vi "ElephantMultThread.vi"   [LabVIEW 2014]
uses:
  <vilib>/NXT/Block Support/NXT_ButtonSelector.ctl
  <vilib>/NXT/Block Support/NXT_InputPort.ctl
  <vilib>/NXT/Block Support/NXT_OutputPort.ctl
  <vilib>/NXT/Dual Mode Library/Waits/Wait_EV3_Color_Red_Less.vi
  <vilib>/NXT/Dual Mode Library/Waits/Wait_EV3_Color_Red_Greater.vi
  <vilib>/NXT/Dual Mode Library/Sound/PlaySoundFile.vi
  <vilib>/NXT/Dual Mode Library/Waits/Wait_Btn_Release.vi
  <vilib>/NXT/Dual Mode Library/Waits/Wait_Btn_Press.vi
  <vilib>/NXT/NXTIO Xnodes/NXTIONodeSubVIs/NXTStopMotors.vi
  <vilib>/NXT/NXTIO Xnodes/NXTIONodeSubVIs/NXTMoveMotors.vi
  <vilib>/NXT/Dual Mode Library/Waits/Wait_LetGo.vi
  <vilib>/NXT/Dual Mode Library/Waits/Wait_Touch.vi
  <vilib>/NXT/NXTIO Xnodes/NXTIONodeSubVIs/LEGOResetMotors.vi
  <vilib>/NXT/NXTIO Xnodes/AddressXNode/NXTIOAddress.xnode
  <vilib>/NXT/NXTIO Xnodes/NXTIOXNode/NXTIO.xnode
  <vilib>/NXT/Subs/LVHSConnector.ctl
  <vilib>/NXT/LegoClasses/BrickReference/BrickReference.lvclass
types:
  T1 = typedef "NXT_InputPort.ctl" = u32
  T2 = typedef "NXT_ButtonSelector.ctl" = u16
  T3 = typedef "NXT_OutputPort.ctl" = u8
  T4 = typedef "LVHSConnector.ctl" = refnum<class "BrickReference.lvclass">
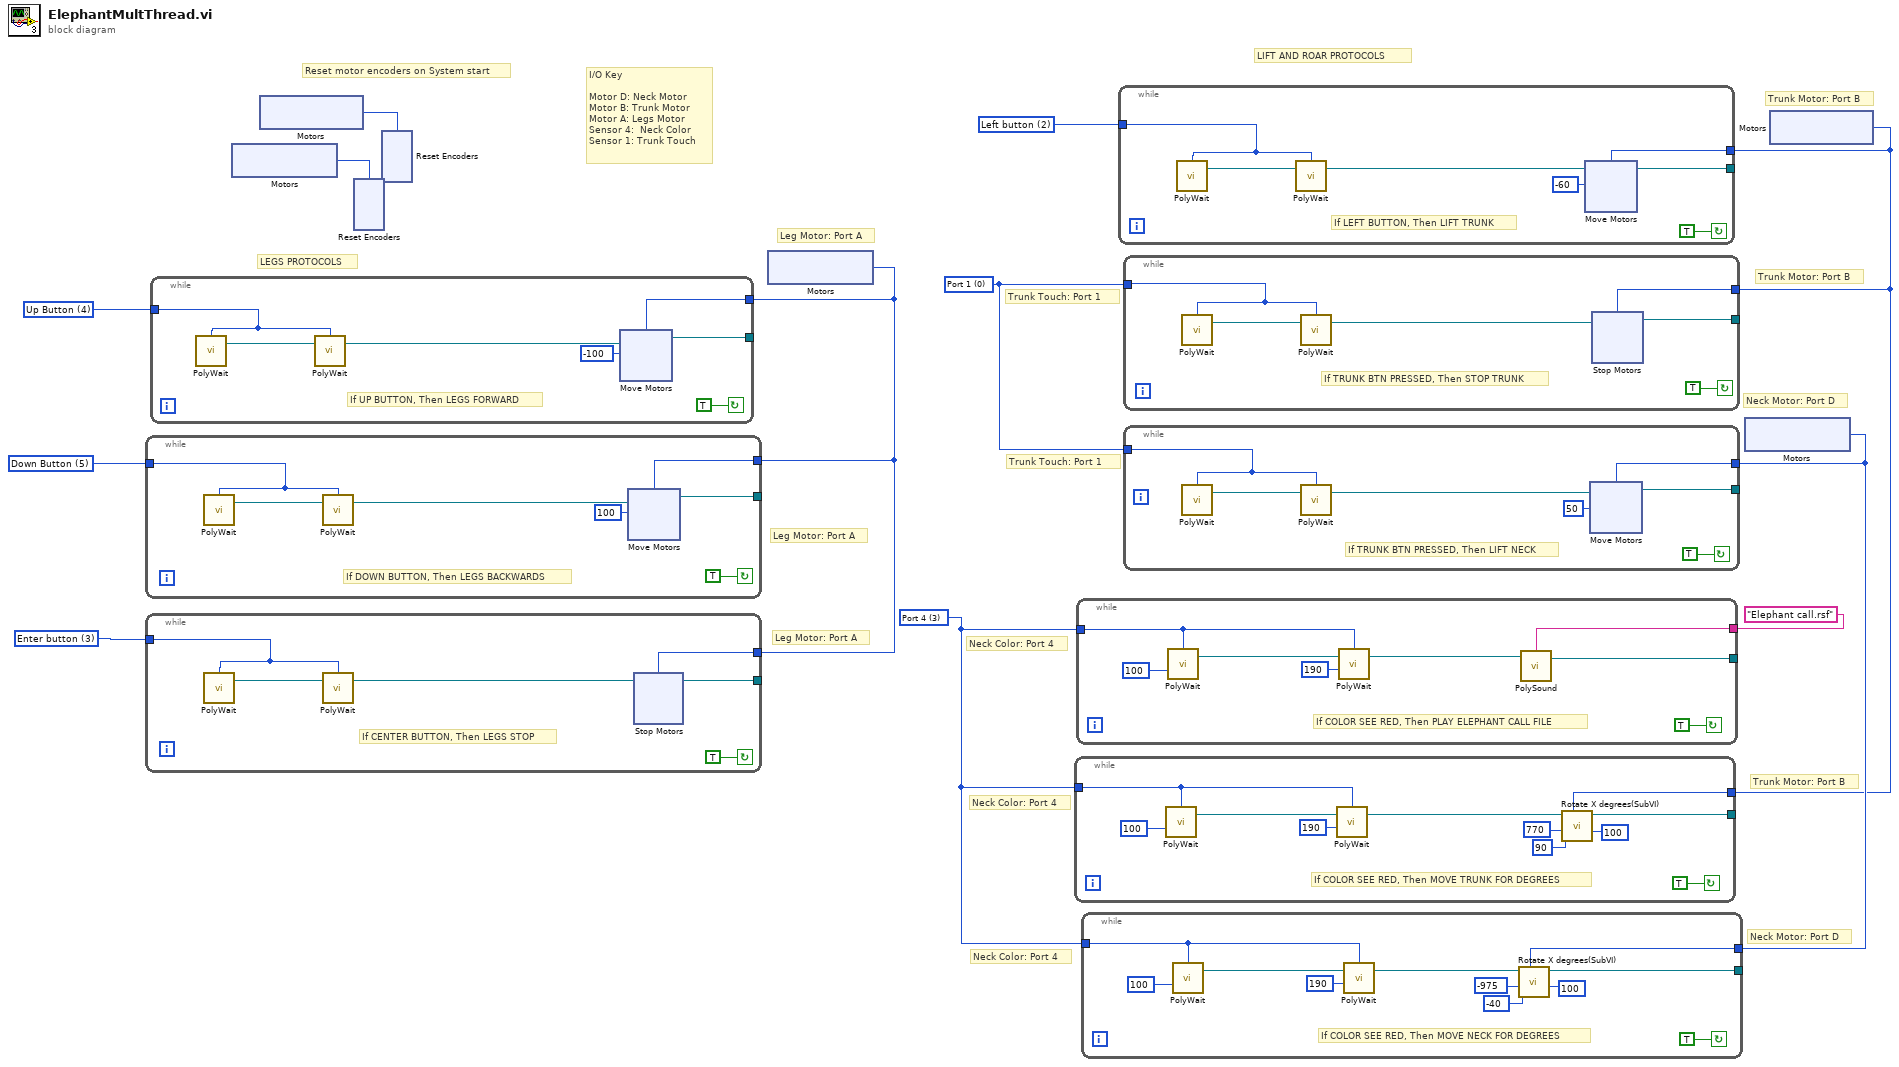
[diagram p0: block diagram]
diagram:
  w1 = T1 3 items=["Port 1", "Port 2", "Port 3", "Port 4"] ("Port (Port 1)")
  w8 = T1 0 items=["Port 1", "Port 2", "Port 3", "Port 4"] ("Port (Port 1)")
  w4 = T2 2 items=["Enter button"=3, "Left button"=2, "Right button"=1, "Up Button"=4, "Down Button"=5] ("Button (Enter button)")
  w9 = T2 3 items=["Enter button"=3, "Left button"=2, "Right button"=1, "Up Button"=4, "Down Button"=5] ("Button (Enter button)")
  w10 = T2 5 items=["Enter button"=3, "Left button"=2, "Right button"=1, "Up Button"=4, "Down Button"=5] ("Button (Enter button)")
  w11 = T2 4 items=["Enter button"=3, "Left button"=2, "Right button"=1, "Up Button"=4, "Down Button"=5] ("Button (Enter button)")
  # "LIFT AND ROAR PROTOCOLS"
  # "Trunk Motor: Port B"
  # "Neck Color: Port 4"
  # "Neck Color: Port 4"
  # "Reset motor encoders on System start"
  # "Trunk Touch: Port 1"
  # "Leg Motor: Port A"
  # "Leg Motor: Port A"
  # "Trunk Motor: Port B"
  # "Neck Motor: Port D"
  # "Neck Color: Port 4"
  # "Trunk Touch: Port 1"
  # "Neck Motor: Port D"
  # "Trunk Motor: Port B"
  # "LEGS PROTOCOLS"
  # "Leg Motor: Port A"
  # "I/O Key\n\nMotor D: Neck Motor\nMotor B: Trunk Motor\nMotor A: Legs Motor\nSensor 4:  Neck Color\nSensor 1: Trunk Touch"
  n1 = xnode "Motors"() -> ("Motor"=w6:T3)
  n2 = xnode "Motors"() -> ("Motor"=w5:T3)
  n3 = xnode "Reset Encoders"("Motors"=w6) -> ()  [unwired: 1 in, 1 out]
  n4 = xnode "Reset Encoders"("Motors"=w5) -> ()  [unwired: 1 in, 1 out]
  n5 = xnode "Motors"() -> ("Motor"=w12:T3)
  n6 = while {
    tunnel: [w17] -> _
    tunnel: w12 -> [w14]
    tunnel: w10 -> [w13]
    stop <- TRUE continue-if-true
    # "If DOWN BUTTON, Then LEGS BACKWARDS"
    n7 = call-poly <vilib>:"PolyWait.vi"("Button (Enter button)"=w13) -> ("NXT/EV3"=w15:T4)  [unwired: 3 in]
    n8 = call-poly <vilib>:"PolyWait.vi"("NXT/EV3"=w15, "Button (Enter button)"=w13) -> ("NXT/EV3"=w18:T4)  [unwired: 2 in]
    n9 = xnode "Move Motors"("Power/Speed 1"=i8 100, "Motors"=w14, "NXT/EV3"=w18) -> ("NXT/EV3"=w17:T4)
  }
  n10 = while {
    tunnel: [w27] -> _
    tunnel: w12 -> [w29]
    tunnel: w9 -> [w28]
    stop <- TRUE continue-if-true
    # "If CENTER BUTTON, Then LEGS STOP"
    n11 = call-poly <vilib>:"PolyWait.vi"("Button (Enter button)"=w28) -> ("NXT/EV3"=w31:T4)  [unwired: 3 in]
    n12 = call-poly <vilib>:"PolyWait.vi"("NXT/EV3"=w31, "Button (Enter button)"=w28) -> ("NXT/EV3"=w30:T4)  [unwired: 2 in]
    n13 = xnode "Stop Motors"("Motors"=w29, "NXT/EV3"=w30) -> ("NXT/EV3"=w27:T4)
  }
  n14 = while {
    tunnel: [w42] -> _
    tunnel: w12 -> [w39]
    tunnel: w11 -> [w38]
    stop <- TRUE continue-if-true
    # "If UP BUTTON, Then LEGS FORWARD"
    n15 = call-poly <vilib>:"PolyWait.vi"("Button (Enter button)"=w38) -> ("NXT/EV3"=w40:T4)  [unwired: 3 in]
    n16 = call-poly <vilib>:"PolyWait.vi"("NXT/EV3"=w40, "Button (Enter button)"=w38) -> ("NXT/EV3"=w43:T4)  [unwired: 2 in]
    n17 = xnode "Move Motors"("Power/Speed 1"=i8 -100, "Motors"=w39, "NXT/EV3"=w43) -> ("NXT/EV3"=w42:T4)
  }
  n18 = while {
    tunnel: [w58] -> _
    tunnel: w1 -> [w53]
    tunnel: "Elephant call.rsf" ("Filename (*.rso/*.rsf)") -> [w52]
    stop <- TRUE continue-if-true
    # "If COLOR SEE RED, Then PLAY ELEPHANT CALL FILE"
    n19 = call-poly <vilib>:"PolyWait.vi"("Red Value (100)"=u8 100, "Port (Port 1)"=w53) -> ("NXT/EV3"=w55:T4)  [unwired: 2 in]
    n20 = call-poly <vilib>:"PolyWait.vi"("Red Value (200)"=u8 190, "NXT/EV3"=w55, "Port (Port 1)"=w53) -> ("NXT/EV3"=w54:T4)  [unwired: 1 in]
    n21 = call-poly <vilib>:"PolySound.vi"("NXT/EV3"=w54, "Filename (*.rso/*.rsf)"=w52) -> ("NXT/EV3"=w58:T4)  [unwired: 2 in]
  }
  n22 = xnode "Motors"() -> ("Motor"=w7:T3)
  n23 = while {
    tunnel: w7 -> [w62]
    tunnel: w1 -> [w66]
    tunnel: [w60] -> _
    stop <- TRUE continue-if-true
    # "If COLOR SEE RED, Then MOVE NECK FOR DEGREES"
    n24 = call-poly <vilib>:"PolyWait.vi"("Red Value (100)"=u8 100, "Port (Port 1)"=w66) -> ("NXT/EV3"=w67:T4)  [unwired: 2 in]
    n25 = call-poly <vilib>:"PolyWait.vi"("Red Value (200)"=u8 190, "NXT/EV3"=w67, "Port (Port 1)"=w66) -> ("NXT/EV3"=w61:T4)  [unwired: 1 in]
    n26 = call "Rotate X degrees(SubVI).vi"("Encoder Delay (msec)"=u32 100 ("Encoder Delay (100 msec)"), "Motor (Port A)"=w62, "Power/Speed 1"=i8 -40, "Position Change (180)"=-975, "BrickReference in"=w61) -> ("BrickReference out"=w60:T4)  [unwired: 6 in]
  }
  n27 = while {
    tunnel: [w74] -> _
    tunnel: w7 -> [w72]
    tunnel: w8 -> [w71]
    stop <- TRUE continue-if-true
    # "If TRUNK BTN PRESSED, Then LIFT NECK"
    n28 = call-poly <vilib>:"PolyWait.vi"("Port (Port 1)"=w71) -> ("NXTEV3"=w76:T4)  [unwired: 3 in]
    n29 = call-poly <vilib>:"PolyWait.vi"("NXT/EV3"=w76, "Port (Port 1)"=w71) -> ("NXT/EV3"=w75:T4)  [unwired: 2 in]
    n30 = xnode "Move Motors"("Power/Speed 1"=i8 50, "Motors"=w72, "NXT/EV3"=w75) -> ("NXT/EV3"=w74:T4)
  }
  n31 = xnode "Motors"() -> ("Motor"=w2:T3)
  n32 = while {
    tunnel: w2 -> [w90]
    tunnel: w1 -> [w91]
    tunnel: [w85] -> _
    stop <- TRUE continue-if-true
    # "If COLOR SEE RED, Then MOVE TRUNK FOR DEGREES"
    n33 = call-poly <vilib>:"PolyWait.vi"("Red Value (100)"=u8 100, "Port (Port 1)"=w91) -> ("NXT/EV3"=w92:T4)  [unwired: 2 in]
    n34 = call-poly <vilib>:"PolyWait.vi"("Red Value (200)"=u8 190, "NXT/EV3"=w92, "Port (Port 1)"=w91) -> ("NXT/EV3"=w86:T4)  [unwired: 1 in]
    n35 = call "Rotate X degrees(SubVI).vi"("Encoder Delay (msec)"=u32 100 ("Encoder Delay (100 msec)"), "Motor (Port A)"=w90, "Power/Speed 1"=i8 90, "Position Change (180)"=770, "BrickReference in"=w86) -> ("BrickReference out"=w85:T4)  [unwired: 6 in]
  }
  n36 = while {
    tunnel: [w98] -> _
    tunnel: w2 -> [w97]
    tunnel: w4 -> [w96]
    stop <- TRUE continue-if-true
    # "If LEFT BUTTON, Then LIFT TRUNK"
    n37 = call-poly <vilib>:"PolyWait.vi"("Button (Enter button)"=w96) -> ("NXT/EV3"=w101:T4)  [unwired: 3 in]
    n38 = call-poly <vilib>:"PolyWait.vi"("NXT/EV3"=w101, "Button (Enter button)"=w96) -> ("NXT/EV3"=w99:T4)  [unwired: 2 in]
    n39 = xnode "Move Motors"("Power/Speed 1"=i8 -60, "Motors"=w97, "NXT/EV3"=w99) -> ("NXT/EV3"=w98:T4)
  }
  n40 = while {
    tunnel: [w112] -> _
    tunnel: w2 -> [w111]
    tunnel: w8 -> [w110]
    stop <- TRUE continue-if-true
    # "If TRUNK BTN PRESSED, Then STOP TRUNK"
    n41 = call-poly <vilib>:"PolyWait.vi"("Port (Port 1)"=w110) -> ("NXTEV3"=w114:T4)  [unwired: 3 in]
    n42 = call-poly <vilib>:"PolyWait.vi"("NXT/EV3"=w114, "Port (Port 1)"=w110) -> ("NXT/EV3"=w113:T4)  [unwired: 2 in]
    n43 = xnode "Stop Motors"("Motors"=w111, "NXT/EV3"=w113) -> ("NXT/EV3"=w112:T4)
  }
